vi "Set message.vi"(10 "WampMessage MsgPack":refnum<class "WampMessage MsgPack.lvclass">, 11 "RegisteredHandler MsgPack in":refnum<class "RegisteredHandler MsgPack.lvclass">) -> (3 "RegisteredHandler MsgPack out":refnum<class "RegisteredHandler MsgPack.lvclass">)   [LabVIEW 2020, in "wamplv.lvlib" / "RegisteredHandler MsgPack.lvclass"]
uses:
  RegisteredHandler MsgPack.lvclass
  RegisteredHandler MsgPack.lvclass/RegisteredHandler MsgPack.ctl
  SerialisedMessages/MsgPackMessage/WampMessage MsgPack.lvclass
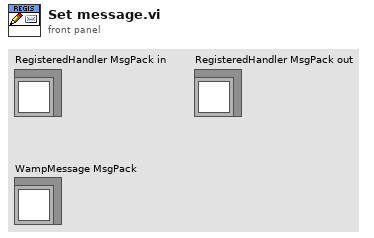
[diagram p1: front panel]
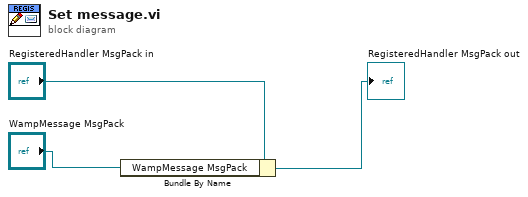
[diagram p0: block diagram]
diagram:
  n1 = Bundle By Name(cluster="RegisteredHandler MsgPack in", "WampMessage MsgPack"="WampMessage MsgPack") -> (→"RegisteredHandler MsgPack out":refnum<class "RegisteredHandler MsgPack.lvclass">)
